vi "FPGA Main.vi"() -> ()   [LabVIEW 2009]
uses:
  <vilib>/Platform/TimedLoop/XDataNode/XDataNode.xnode
  <vilib>/Platform/TimedLoop/XDataNode/loadlvalarms.vi
  <vilib>/Platform/TimedLoop/XDataNode/timing_clust.ctl
  <vilib>/Platform/TimedLoop/XDataNode/nitl_modes.ctl
  <vilib>/Platform/TimedLoop/XDataNode/wakeup.ctl
  <vilib>/eio/EIONode/EIONode.xnode
  <vilib>/rvi/eio/nirviEIOImplementation/nirviEIOImplementation.xnode
  <vilib>/rvi/eio/common/nirviEmuTemplateMethod_noerrors.vi
  <vilib>/rvi/eio/common/nirviEmuClasses.ctl
  <vilib>/Platform/TimedLoop/XDataNode/XDNodeRunTimeDep.lvlib
  <vilib>/NI VeriStand/FPGA/NI_VS FPGA Support.lvlib
panel:
  in  "Start Encoders":bool
  out "Travel dT (Ticks)":u32
  out "Pitch dT (Ticks)":u32
  out "Elevation dT (Ticks)":u32
  out "Travel Set High":u32
  in  "Clock Divider":u16=500
  out "Sensor Ok?":bool
  out "Travel Velocity":i32
  out "Travel Position":i32
  out "ENC 2 In Vel/Acc Update":bool
  out "Pitch Velocity":i32
  out "Pitch Position":i32
  out "ENC 1 In Vel/Acc Update":bool
  out "Elevation Velocity":i32
  out "Elevation Position":i32
  out "ENC 0 In Vel/Acc Update":bool
  in  "ENC In Clock":bool=TRUE
  in  "Fan High Time 2":u32
  in  "Fan High Time 1":u32
  out "Elevation Set High":u32
  in  "PWM Period (ticks)":u32=100000
  # "PWM In"
  # "Configuration"
  # "Internal Controls"
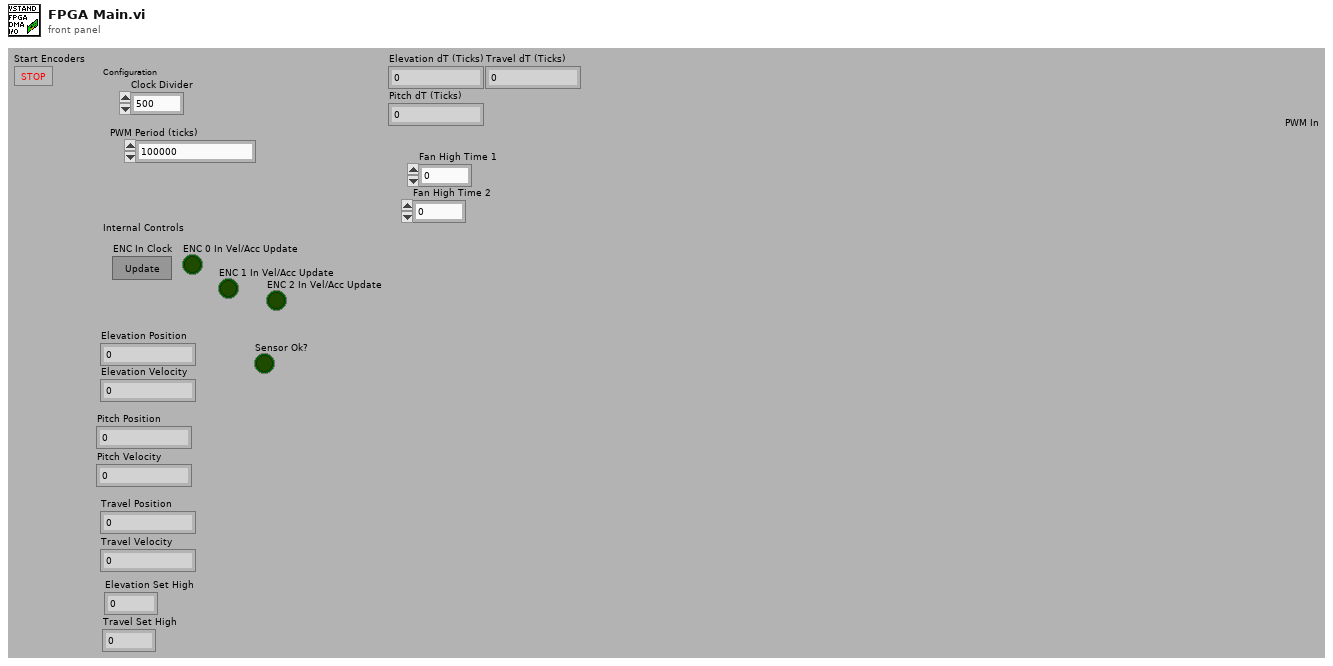
[diagram p1: front panel]
types:
  T1 = typedef "XDNodeRunTimeDep.lvlib/timing_clust.ctl" = cluster{"Expected End [f-1]":u64, "Actual End [f-1]":u64, "Finished Late? [f-1]":bool, "Expected End [i-1]":u64, "Actual End [i-1]":u64, "Finished Late? [i-1]":bool, "Expected Start [i]":u64, "Actual Start [i]":u64, "Expected Start [f]":u64, "Actual Start [f]":u64, "Source Name":string, "Structure Name":string, "Period":i64, "Deadline":i64, "Offset":i64, "Start":i64, "Priority":i32, "Timeout":i32, "Mode":T2, "Wakeup Reason":T3, "Error":errorcluster, "Source Type":string, "Secondary Source Type":string, "Global End Time":u64, "Global Start Time":u64, "Frame Duration":u64, "Iteration Duration":u64, "Assigned CPU":i32, "I/O Scan Engine Mode":u32}
  T2 = typedef "XDNodeRunTimeDep.lvlib/nitl_modes.ctl" = enum32{"No Change", "Process missed periods, maintain original phase", "Discard missed periods, maintain original phase", "Process missed periods, ignore original phase", "Discard missed periods, ignore original phase"}
  T3 = typedef "XDNodeRunTimeDep.lvlib/wakeup.ctl" = enum32{"Normal", "Aborted", "Asynchronous wakeup", "Timing source error", "Timed loop error", "Timeout"}
  T4 = typedef "nirviEmuClasses.ctl" = enum16{"IO Read", "IO Write", "Method", "Property Read", "Property Write"}
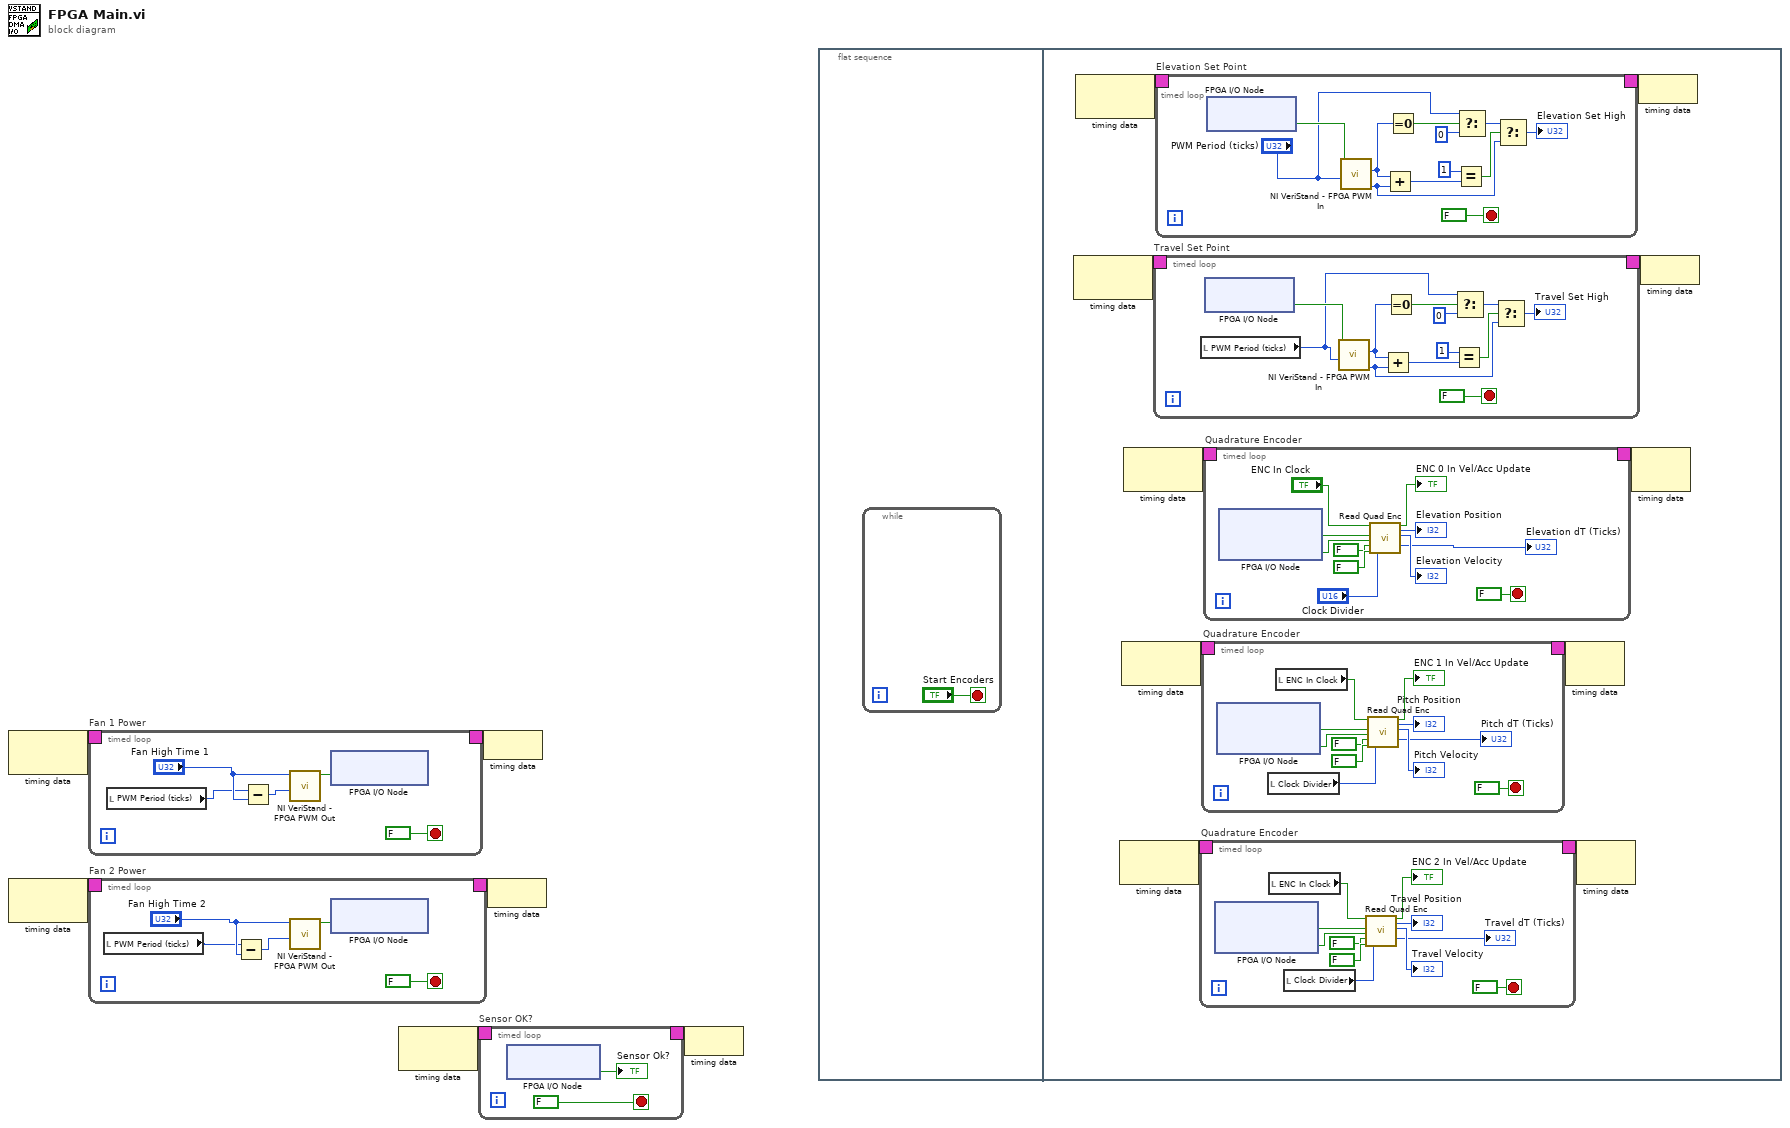
[diagram p0: block diagram]
diagram:
  n1 = node-c288() -> (w6:T1)  [unwired: 1 in]
  n2 = node-c288() -> (w4:T1)  [unwired: 1 in]
  n3 = timed-loop "Fan 1 Power" {
    timing: w6 -> [_]
    timing-out: [_] -> w5
    stop <- FALSE stop-if-true
    n4 = local read "PWM Period (ticks)"() -> (w7:u32)
    n5 = Subtract(x=w7, y="Fan High Time 1") -> (x-y=w9:u32)
    n6 = call <vilib>:"NI VeriStand - FPGA PWM Out.vi"("_Low Time"=w9, "_High Time"="Fan High Time 1") -> ("Output"=w10:bool)  [unwired: 9 in]
    n7 = xnode "FPGA I/O Node"("PWM 2 Out"=w10) -> ()  [unwired: 1 in, 1 out]
  }
  n8 = timed-loop "Fan 2 Power" {
    timing: w4 -> [_]
    timing-out: [_] -> w3
    stop <- FALSE stop-if-true
    n9 = local read "PWM Period (ticks)"() -> (w25:u32)
    n10 = Subtract(x=w25, y="Fan High Time 2") -> (x-y=w26:u32)
    n11 = call <vilib>:"NI VeriStand - FPGA PWM Out.vi"("_Low Time"=w26, "_High Time"="Fan High Time 2") -> ("Output"=w28:bool)  [unwired: 9 in]
    n12 = xnode "FPGA I/O Node"("PWM 3 Out"=w28) -> ()  [unwired: 1 in, 1 out]
  }
  n13 = node-c288() -> (w2:T1)  [unwired: 1 in]
  n14 = timed-loop "Sensor OK?" {
    timing: w2 -> [_]
    timing-out: [_] -> w1
    stop <- FALSE stop-if-true
    n15 = xnode "FPGA I/O Node"() -> ("Sensor OK"=→"Sensor Ok?":bool)  [unwired: 1 in, 1 out]
  }
  n16 = node-c288(w5) -> ()
  n17 = node-c288(w3) -> ()
  n18 = node-c288(w1) -> ()
  n19 = flat-sequence {
    frame #0 {
      n20 = while {
        stop <- "Start Encoders" stop-if-true
      }
    }
    frame #1 {
      n21 = node-c288() -> (w68:T1)  [unwired: 1 in]
      n22 = node-c288() -> (w76:T1)  [unwired: 1 in]
      n23 = node-c288() -> (w70:T1)  [unwired: 1 in]
      n24 = node-c288() -> (w72:T1)  [unwired: 1 in]
      n25 = node-c288() -> (w74:T1)  [unwired: 1 in]
      n26 = timed-loop "Travel Set Point" {
        timing: w68 -> [_]
        timing-out: [_] -> w67
        stop <- FALSE stop-if-true
        n27 = local read "PWM Period (ticks)"() -> (w77:u32)
        n28 = xnode "FPGA I/O Node"() -> ("PWM 1 In"=w87:bool)  [unwired: 1 in, 1 out]
        n29 = call <vilib>:"NI VeriStand - FPGA PWM In.vi"("Time Out"=w77, "Value"=w87) -> ("High time"=w83:u32, "Low Time"=w81:u32)  [unwired: 8 in]
        n30 = Add(x=w81, y=w83) -> (x+y=w86:u32)
        n31 = Equal To 0?(x=w81) -> (x = 0?=w82:bool)
        n32 = Equal?(x=u32 1, y=w86) -> (x = y?=w84:bool)
        n33 = Select(t=w77, s=w82, f=u32 0) -> (s? t:f=w79:u32)
        n34 = Select(t=w79, s=w84, f=w83) -> (s? t:f=→"Travel Set High":u32)
      }
      n35 = timed-loop "Elevation Set Point" {
        timing: w76 -> [_]
        timing-out: [_] -> w75
        stop <- FALSE stop-if-true
        n36 = xnode "FPGA I/O Node"() -> ("PWM 0 In"=w281:bool)  [unwired: 1 in, 1 out]
        n37 = call <vilib>:"NI VeriStand - FPGA PWM In.vi"("Time Out"="PWM Period (ticks)", "Value"=w281) -> ("High time"=w277:u32, "Low Time"=w275:u32)  [unwired: 8 in]
        n38 = Add(x=w275, y=w277) -> (x+y=w280:u32)
        n39 = Equal To 0?(x=w275) -> (x = 0?=w276:bool)
        n40 = Equal?(x=u32 1, y=w280) -> (x = y?=w278:bool)
        n41 = Select(t="PWM Period (ticks)", s=w276, f=u32 0) -> (s? t:f=w273:u32)
        n42 = Select(t=w273, s=w278, f=w277) -> (s? t:f=→"Elevation Set High":u32)
      }
      n43 = timed-loop "Quadrature Encoder" {
        timing: w70 -> [_]
        timing-out: [_] -> w69
        stop <- FALSE ("stop") stop-if-true
        n44 = xnode "FPGA I/O Node"() -> ("ENC 2 A+ In"=w117:bool, "ENC 2 B+ In"=w116:bool)  [unwired: 2 in, 2 out]
        n45 = local read "ENC In Clock"() -> (w114:bool)
        n46 = local read "Clock Divider"() -> (w113:u16)
        n47 = call "Read Quad Enc.vi"("Clock"=w114, "A"=w117, "B"=w116, "Z"=FALSE, "Polarity"=FALSE, "Clock Divider"=w113) -> ("Vel/Acc Update"=→"ENC 2 In Vel/Acc Update":bool, "Position (Counts)"=→"Travel Position":i32, "Velocity (Counts/Interval)"=→"Travel Velocity":i32, "dT (Ticks)"=→"Travel dT (Ticks)":u32)  [unwired: 2 in, 8 out]
      }
      n48 = timed-loop "Quadrature Encoder" {
        timing: w72 -> [_]
        timing-out: [_] -> w71
        stop <- FALSE ("stop") stop-if-true
        n49 = xnode "FPGA I/O Node"() -> ("ENC 1 A+ In"=w170:bool, "ENC 1 B+ In"=w169:bool)  [unwired: 2 in, 2 out]
        n50 = local read "Clock Divider"() -> (w166:u16)
        n51 = local read "ENC In Clock"() -> (w167:bool)
        n52 = call "Read Quad Enc.vi"("Clock"=w167, "A"=w170, "B"=w169, "Z"=FALSE, "Polarity"=FALSE, "Clock Divider"=w166) -> ("Vel/Acc Update"=→"ENC 1 In Vel/Acc Update":bool, "Position (Counts)"=→"Pitch Position":i32, "Velocity (Counts/Interval)"=→"Pitch Velocity":i32, "dT (Ticks)"=→"Pitch dT (Ticks)":u32)  [unwired: 2 in, 8 out]
      }
      n53 = timed-loop "Quadrature Encoder" {
        timing: w74 -> [_]
        timing-out: [_] -> w73
        stop <- FALSE ("stop") stop-if-true
        n54 = xnode "FPGA I/O Node"() -> ("ENC 0 A+ In"=w223:bool, "ENC 0 B+ In"=w222:bool)  [unwired: 2 in, 2 out]
        n55 = call "Read Quad Enc.vi"("Clock"="ENC In Clock", "A"=w223, "B"=w222, "Z"=FALSE, "Polarity"=FALSE, "Clock Divider"="Clock Divider") -> ("Vel/Acc Update"=→"ENC 0 In Vel/Acc Update":bool, "Position (Counts)"=→"Elevation Position":i32, "Velocity (Counts/Interval)"=→"Elevation Velocity":i32, "dT (Ticks)"=→"Elevation dT (Ticks)":u32)  [unwired: 2 in, 8 out]
      }
      n56 = node-c288(w71) -> ()  [unwired: 1 out]
      n57 = node-c288(w69) -> ()  [unwired: 1 out]
      n58 = node-c288(w73) -> ()  [unwired: 1 out]
      n59 = node-c288(w75) -> ()
      n60 = node-c288(w67) -> ()
    }
  }
